vi "Filtering Signals.vi"() -> ()   [LabVIEW 2023]
panel:
  out "Waveform Chart":dynamicdata(graph)
  in  "Frequency(Hz)":dbl(slide) scale=0.0..100.0
  in  "Stop Button":bool
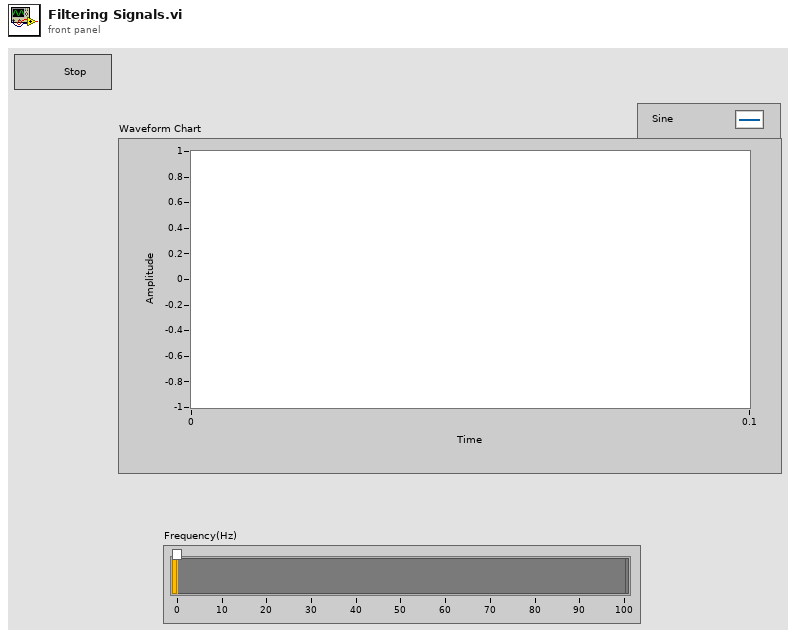
[diagram p1: front panel]
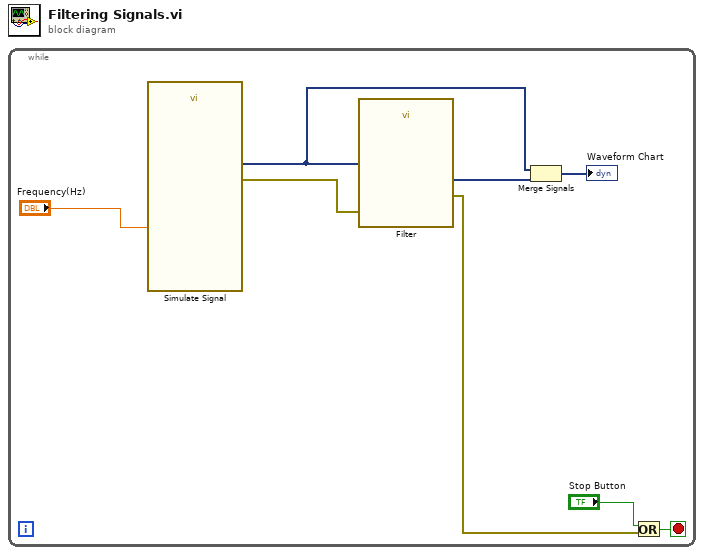
[diagram p0: block diagram]
diagram:
  n1 = while {
    stop <- w8 stop-if-true
    n2 = call "Simulate Signal"("Frequency"="Frequency(Hz)") -> ("Sine"=w1:dynamicdata, "error out"=w7:errorcluster)  [unwired: 13 in]
    n3 = call "Filter"("error in (no error)"=w7, "Signal"=w1) -> ("error out"=w6:errorcluster, "Filtered Signal"=w2:dynamicdata)  [unwired: 8 in]
    n4 = Merge Signals(w1, w2) -> (→"Waveform Chart":dynamicdata)
    n5 = Or(x="Stop Button", y=w6) -> (x .or. y?=w8:bool)
  }
